vi "Periodic Tasks.vi"   [LabVIEW 2013]
doc: "This VI runs in parallel to other tasks. It can contain as many user-defined periodic loops as you need. These can carry out PID or other sorts of timed response."
uses:
  <vilib>/Rock Robotics/SystemInterfaces/Utilities/FPGA_UtilitiesLED State.ctl
  <vilib>/Rock Robotics/SystemInterfaces/Utilities/FPGA_UtilitiesLED Source.ctl
  <vilib>/Rock Robotics/WPI/Compressor/WPI_CompressorGetSetRefNum.vi
  Robot Global Data.vi
types:
  T1 = typedef "FPGA_UtilitiesLED Source.ctl" = enum16{"User LED", "FPGA LED"}
  T2 = typedef "FPGA_UtilitiesLED State.ctl" = enum16{"Off", "On", "Toggle"}
  T3 = typedef "WPI_CompressorDevRef.ctl" = cluster{"DevStatus":errorcluster, "DigitalInputDevRef":T4, "RelayDevRef":T7}
  T4 = typedef "WPI_DigitalInputDevRef.ctl" = cluster{"DevStatus":errorcluster, "DIO Channel":T5, "Digital Module":T6}
  T5 = typedef "FPGA_DIOChannel.ctl" = enum8{"DIO 1", "DIO 2", "DIO 3", "DIO 4", "DIO 5", "DIO 6", "DIO 7", "DIO 8", "DIO 9", "DIO 10", "DIO 11", "DIO 12", "DIO 13", "DIO 14", "Invalid"}
  T6 = typedef "FPGA_TypedefDigitalModule.ctl" = enum16{"Digital Module 1", "Digital Module 2"}
  T7 = typedef "WPI_RelayDevRef.ctl" = cluster{"DevStatus":errorcluster, "Relay Channel":T8, "Digital Module":T6, "Relay Direction":T9}
  T8 = typedef "FPGA_DIORelayChannel.ctl" = enum8{"Relay 1", "Relay 2", "Relay 3", "Relay 4", "Relay 5", "Relay 6", "Relay 7", "Relay 8", "Invalid"}
  T9 = typedef "WPI_RelayDirection.ctl" = enum16{"Both directions", "Forward only", "Reverse only"}
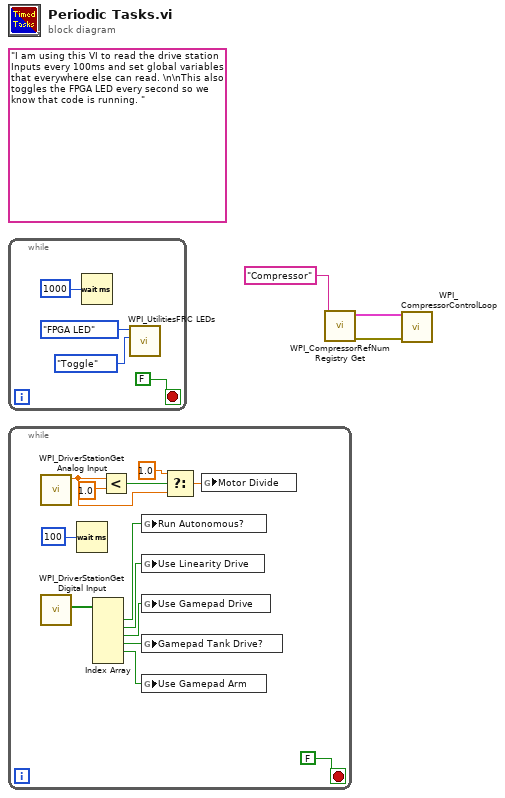
[diagram p0: block diagram]
diagram:
  (unwired) "I am using this VI to read the drive station Inputs every 100ms and set global variables that everywhere else can read. \n\nThis also toggles the FPGA LED every second so we know that code is running. "
  n1 = while {
    stop <- FALSE stop-if-true
    n2 = Wait (ms)(milliseconds to wait=u32 1000) -> ()  [unwired: 1 out]
    n3 = call <vilib>:"WPI_UtilitiesFRC LEDs.vi"("State"=FPGA_UtilitiesLED_State."Toggle", "LED Type"=FPGA_UtilitiesLED_Source."FPGA LED") -> ()  [unwired: 1 in, 9 out]
  }
  n4 = while {
    stop <- FALSE stop-if-true
    n5 = call <vilib>:"WPI_DriverStationGet Analog Input.vi"() -> ("Analog 1 (V)"=w14:dbl)  [unwired: 11 out]
    n6 = call <vilib>:"WPI_DriverStationGet Digital Input.vi"() -> ("Driver Station Digital Input (1-8)"=w18:bool[])  [unwired: 11 out]
    n7 = Wait (ms)(milliseconds to wait=u32 100) -> ()  [unwired: 1 out]
    n8 = Index Array(array=w18) -> (element #1=w12:bool, element #2=w10:bool, element #3=w11:bool, element #4=w9:bool, element #5=w8:bool)  [unwired: 6 in, 1 out]
    n9 = Less?(x=w14, y=1.0) -> (x < y?=w16:bool)
    n10 = global write "Robot Global Data.vi" "Run Autonomous?"(w12) -> ()
    n11 = global write "Robot Global Data.vi" "Use Linearity Drive"(w10) -> ()
    n12 = global write "Robot Global Data.vi" "Use Gamepad Drive"(w11) -> ()
    n13 = global write "Robot Global Data.vi" "Gamepad Tank Drive?"(w9) -> ()
    n14 = global write "Robot Global Data.vi" "Use Gamepad Arm"(w8) -> ()
    n15 = Select(t=1.0, s=w16, f=w14) -> (s? t:f=w13:dbl)
    n16 = global write "Robot Global Data.vi" "Motor Divide"(w13) -> ()
  }
  n17 = call <vilib>:"WPI_CompressorRefNum Registry Get.vi"("refnum name"="Compressor") -> ("error out"=w1:errorcluster, "CompressorDevRef"=w3:T3)  [unwired: 9 in]
  n18 = call <vilib>:"WPI_CompressorControlLoop.vi"("error in (no error)"=w1, "CompressorDevRef"=w3) -> ()  [unwired: 10 in]
